vi "获取时间日期.vi"(0 "布尔 2":bool) -> (1 "时间":string, 2 "日期":string)   [LabVIEW 2016]
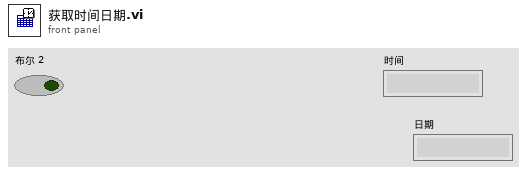
[diagram p1: front panel]
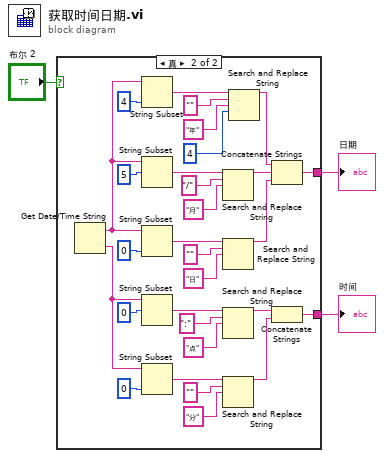
[diagram p0: block diagram]
diagram:
  n1 = case shown="真" "布尔 2" {
    tunnel: [_ w5] -> w2
    tunnel: [_ w4] -> w1
    frame False {
    }
    frame True {
      n2 = Get Date/Time String() -> (date string=w10:string, time string=w9:string)  [unwired: 3 in]
      n3 = String Subset(string=w10, length (rest)=4 ("长度（剩余）")) -> (substring=w23:string)  [unwired: 1 in]
      n4 = String Subset(string=w10, offset (0)=5 ("长度（剩余）")) -> (substring=w17:string)  [unwired: 1 in]
      n5 = String Subset(string=w10, length (rest)=0 ("长度（剩余）")) -> (substring=w6:string)  [unwired: 1 in]
      n6 = String Subset(string=w9, offset (0)=0 ("长度（剩余）")) -> (substring=w7:string)  [unwired: 1 in]
      n7 = String Subset(string=w9, length (rest)=0 ("长度（剩余）")) -> (substring=w8:string)  [unwired: 1 in]
      n8 = Search and Replace String(input string=w17, search string="/" ("搜索字符串"), replace string="月" ("搜索字符串")) -> (result string=w32:string)  [unwired: 5 in, 3 out]
      n9 = Search and Replace String(input string=w6, search string="" ("搜索字符串"), replace string="日" ("搜索字符串")) -> (result string=w31:string)  [unwired: 5 in, 3 out]
      n10 = Search and Replace String(input string=w7, search string=":" ("搜索字符串"), replace string="点" ("搜索字符串")) -> (result string=w30:string)  [unwired: 5 in, 3 out]
      n11 = Search and Replace String(input string=w8, search string="" ("搜索字符串"), replace string="分" ("搜索字符串")) -> (result string=w29:string)  [unwired: 5 in, 3 out]
      n12 = Search and Replace String(input string=w23, search string="" ("搜索字符串"), replace string="年" ("搜索字符串"), offset=4 ("长度（剩余）")) -> (result string=w33:string)  [unwired: 4 in, 3 out]
      n13 = Concatenate Strings(w33, w32, w31) -> (w5:string)
      n14 = Concatenate Strings(w30, w29) -> (w4:string)
    }
  }
  "日期" <- w2
  "时间" <- w1
